vi "OP80_Data.vi"() -> (0 "OP80_DATECODE":T1)   [LabVIEW 2020]
uses:
  Controls/OP80_DataCluster.ctl
panel:
  out "[CT]":dbl
  out "OP80_014_FINAL_VIEWING":T2
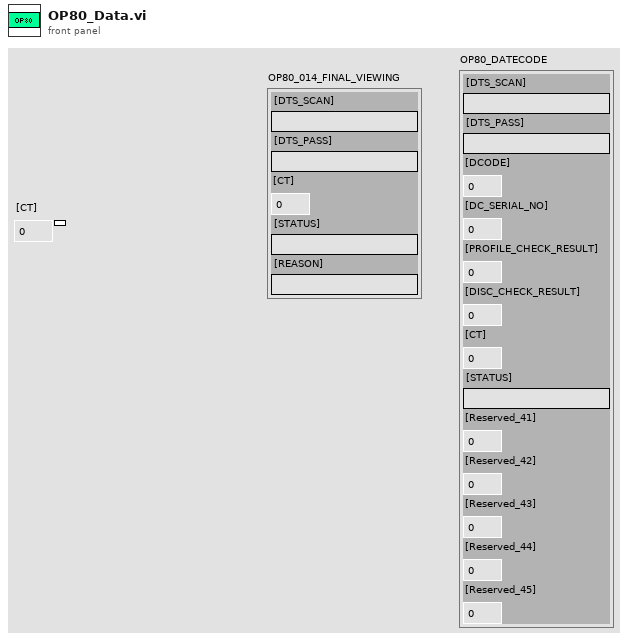
[diagram p1: front panel]
types:
  T1 = cluster{"[DTS_SCAN]":string, "[DTS_PASS]":string, "[DCODE]":dbl, "[DC_SERIAL_NO]":dbl, "[PROFILE_CHECK_RESULT]":dbl, "[DISC_CHECK_RESULT]":dbl, "[CT]":dbl, "[STATUS]":string, "[Reserved_41]":dbl, "[Reserved_42]":dbl, "[Reserved_43]":dbl, "[Reserved_44]":dbl, "[Reserved_45]":dbl}
  T2 = typedef "OP80_DataCluster.ctl" = cluster{"[DTS_SCAN]":string, "[DTS_PASS]":string, "[CT]":dbl, "[STATUS]":string, "[REASON]":string}
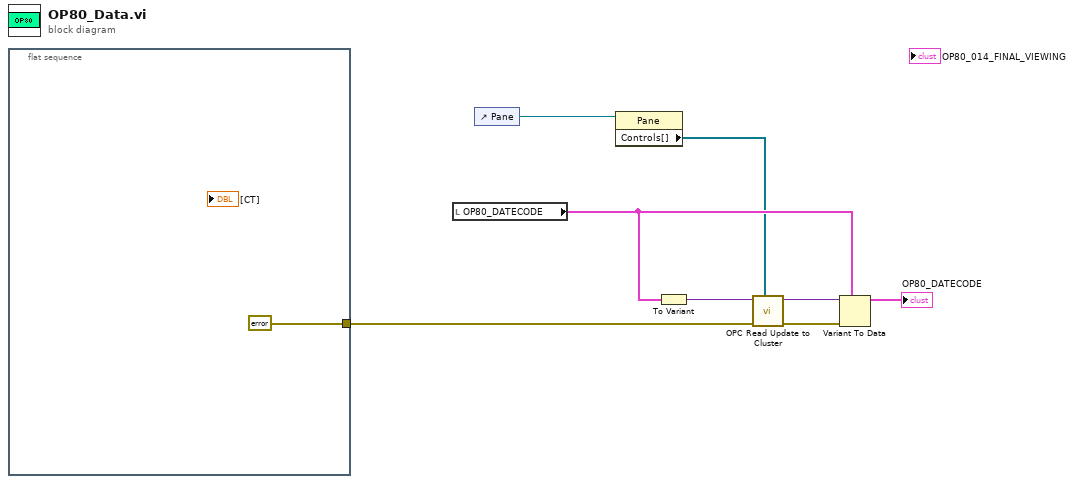
[diagram p0: block diagram]
diagram:
  n1 = flat-sequence {
    tunnel: [errorcluster {"status"=FALSE, "code"=0, "source"=""} ("error in (no error)")] -> w4
    frame #0 {
    }
  }
  n2 = local read "OP80_DATECODE"() -> (w5:T1)
  n3 = control-ref of="Pane"() -> (w3:refnum<vi>)
  n4 = property class="Pane"(reference=w3) -> ("Controls[]"=w2:refnum<vi>[])  [unwired: 1 in, 2 out]
  n5 = To Variant(anything=w5) -> (Variant=w6:variant)
  n6 = call "OPC Read Update to Cluster.vi"("Controls[]"=w2, "error in (no error)"=w4, "Variant in"=w6) -> ("error out"=w7:errorcluster, "Variant out"=w8:variant)  [unwired: 7 in]
  n7 = Variant To Data(error in=w7, type=w5, Variant=w8) -> (data=→"OP80_DATECODE":T1)  [unwired: 1 out]
